vi "Check volume free space.vi"(8 "error in":errorcluster, 10 "Bytes to copy":i64, 11 "path":path=path "c:/") -> (0 "error out":errorcluster, 1 "Volume string":string, 2 "%Memory full":dbl, 3 "path out":path, 4 "Volume Valid?":bool, 5 "Full?":bool)   [LabVIEW 2013, in "FileIO lib.lvlib"]
uses:
  FileIO lib.lvlib
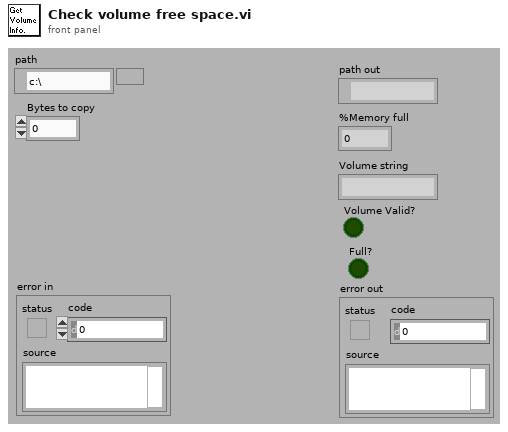
[diagram p1: front panel]
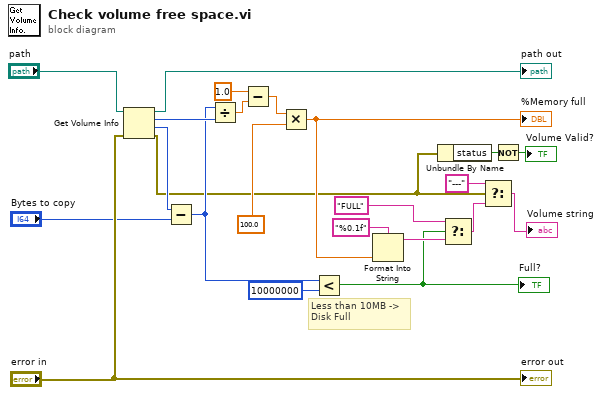
[diagram p0: block diagram]
diagram:
  # "Less than 10MB ->\nDisk Full"
  n1 = Get Volume Info(8:"error in", 11:"path") -> (0:w3:errorcluster, 1:w8:i64, 2:w22:i64, 3:→"path out":path)  [unwired: 2 out]
  n2 = Subtract(x=w8, y="Bytes to copy") -> (x-y=w6:i64)
  n3 = Divide(x=w6, y=w22) -> (x/y=w11:dbl)
  n4 = Subtract(x=1.0, y=w11) -> (x-y=w9:dbl)
  n5 = Multiply(x=w9, y=100.0) -> (x*y=w19:dbl)
  "%Memory full" <- w19
  n6 = Less?(x=w6, y=i64 10000000) -> (x < y?=w4:bool)
  "Full?" <- w4
  n7 = Format Into String(format string="%0.1f", w19) -> (resulting string=w17:string)  [unwired: 2 in, 1 out]
  n8 = Unbundle By Name(w3) -> ("status"=w2:bool)
  n9 = Select(t="FULL", s=w4, f=w17) -> (s? t:f=w14:string)
  n10 = Select(t="---", s=w3, f=w14) -> (s? t:f=→"Volume string":string)
  n11 = Not(x=w2) -> (.not. x?=→"Volume Valid?":bool)
  "error out" <- "error in"
